vi "Set File Ref.vi"(8 "error in":errorcluster, 10 "File Ref":refnum<file>, 11 "FileHandler in":refnum<class "FileHandler.lvclass">) -> (0 "error out":errorcluster, 3 "FileHandler out":refnum<class "FileHandler.lvclass">)   [LabVIEW 2024, in "hse-logger.lvlib" / "FileHandler.lvclass"]
doc: "____\nHAMPEL SOFTWARE ENGINEERING v2.2.2 (2025-01-16 15:41)"
uses:
  <vilib>/Hampel Software Engineering/HSE Logger/Handler/FileHandler/FileHandler.lvclass
  <vilib>/Hampel Software Engineering/HSE Logger/Handler/FileHandler/FileHandler.lvclass/FileHandler.ctl
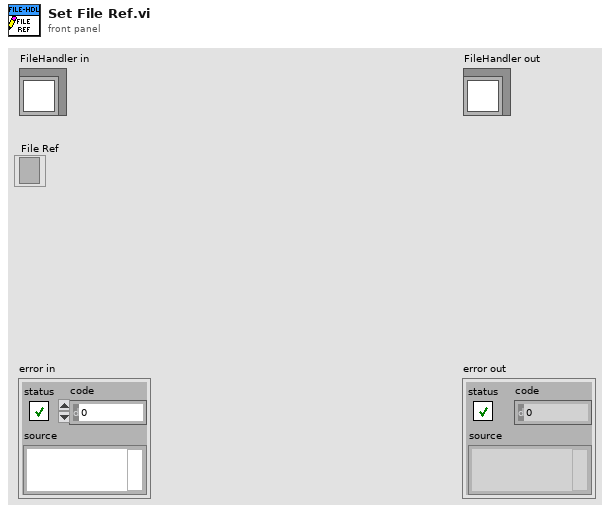
[diagram p1: front panel]
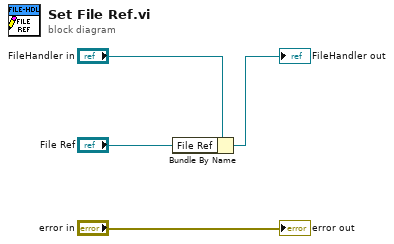
[diagram p0: block diagram]
diagram:
  n1 = Bundle By Name(cluster="FileHandler in", "File Ref"="File Ref") -> (→"FileHandler out":refnum<class "FileHandler.lvclass">)
  "error out" <- "error in"
